vi "TSM Initialise Global (Main Sequence).vi"(0 "TSM context":T1) -> (15 "error out":errorcluster)   [LabVIEW 2019]
uses:
  <vilib>/NI_TestStand_SemiconductorModule/NI_TestStand_Semiconductor_Module.lvlibp/PinMap/General/SemiconductorModuleContext.ctl
  Common/Instrument Control/DCPower/TSM/TSM SSC DCPower.ctl
  <vilib>/NI_TestStand_SemiconductorModule/NI_TestStand_Semiconductor_Module.lvlibp/PinMap/PinQueryContext/MultiplePinMultipleSessionQueryContext/MultiplePinMultipleSessionQueryContext.lvclass
  Common/Instrument Control/DCPower/SSC DCPower/SSC DCPower.ctl
  Common/Instrument Control/Shared SubVIs/TSM Pin Abstraction/TSM Pin Information.ctl
  Common/Instrument Control/Shared SubVIs/TSM Pin Abstraction/TSM Pin Type Identifier.ctl
  Common/Instrument Control/Shared SubVIs/TSM Pin Abstraction/TSM Expanded Pin Information.ctl
  Common/Instrument Control/Relay/Pin Map/TSM Relay.ctl
  Common/Instrument Control/DAQmx/Pin Map/TSM DAQmx Multi-Task.ctl
  Common/Instrument Control/DAQmx/Pin Map/SSC DAQmx.ctl
  TSM Context Data Access/TSM Context Data Access.lvclass/TSM Context Data Access.ctl
  TSM Context Data Access/Public/Properties/D1 - Write.vi
  TSM Context Data Access/Public/Properties/G4 - Write.vi
  TSM Context Data Access/Public/Properties/G8 - Write.vi
  TSM Context Data Access/Public/Properties/G9 - Write.vi
  TSM Context Data Access/Public/Properties/I0 - Write.vi
  TSM Context Data Access/Public/Properties/L - Write.vi
  TSM Context Data Access/Public/Properties/L0 - Write.vi
  TSM Context Data Access/Public/Properties/L1 - Write.vi
  TSM Context Data Access/Public/Properties/L7 - Write.vi
  TSM Context Data Access/Public/Properties/L2 - Write.vi
  TSM Context Data Access/Public/Properties/L3 - Write.vi
  TSM Context Data Access/Public/Properties/L4 - Write.vi
  TSM Context Data Access/Public/Properties/L5 - Write.vi
  TSM Context Data Access/Public/Properties/MODE1 - Write.vi
  TSM Context Data Access/Public/Properties/F0 - Write.vi
  TSM Context Data Access/Public/Properties/F1 - Write.vi
  TSM Context Data Access/Public/Properties/F2 - Write.vi
  TSM Context Data Access/Public/Properties/F3 - Write.vi
  TSM Context Data Access/Public/Properties/F4 - Write.vi
  TSM Context Data Access/Public/Properties/F5 - Write.vi
  TSM Context Data Access/Public/Properties/F7 - Write.vi
  TSM Context Data Access/Public/Properties/F8 - Write.vi
  TSM Context Data Access/Public/Properties/F9 - Write.vi
  TSM Context Data Access/Public/Properties/Q1 - Write.vi
  TSM Context Data Access/Public/Properties/Q2 - Write.vi
  TSM Context Data Access/Public/Properties/Q3 - Write.vi
  TSM Context Data Access/Public/Properties/Q4 - Write.vi
  TSM Context Data Access/Public/Properties/Q5 - Write.vi
  TSM Context Data Access/Public/Properties/Q6 - Write.vi
  TSM Context Data Access/Public/Properties/Q7 - Write.vi
  TSM Context Data Access/Public/Properties/Q8 - Write.vi
  TSM Context Data Access/Public/Properties/Q9 - Write.vi
  TSM Context Data Access/Public/Properties/DNUM - Read.vi
  <vilib>/NI_TestStand_SemiconductorModule/NI_TestStand_Semiconductor_Module.lvlibp/PinMap/Site and Global Data/SetSiteData.vi
  <vilib>/NI_TestStand_SemiconductorModule/NI_TestStand_Semiconductor_Module.lvlibp/PinMap/Site and Global Data/SetGlobalData.vi
  <vilib>/NI_TestStand_SemiconductorModule/NI_TestStand_Semiconductor_Module.lvlibp/PinMap/Site and Global Data/GetGlobalData.vi
  <vilib>/NI_TestStand_SemiconductorModule/NI_TestStand_Semiconductor_Module.lvlibp
  TSM Context Data Access/TSM Context Data Access.lvclass
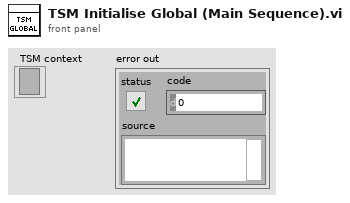
[diagram p1: front panel]
types:
  T1 = typedef "NI_TestStand_Semiconductor_Module.lvlibp/SemiconductorModuleContext.ctl" = refnum<k7>
  T2 = cluster{"unloaded12VRLY":dbl[], "vdiode":dbl[], "RelayDrop":dbl[][]}
  T3 = typedef "TSM SSC DCPower.ctl" = cluster{"Pin Query Context":refnum<class "MultiplePinMultipleSessionQueryContext.lvclass">, "SSC":T4[], "Site Numbers":i32[], "Pins":T5[], "Pins Expanded":T7[]}
  T4 = typedef "SSC DCPower.ctl" = cluster{"Session":refnum<k15>, "Chan":string, "Channel List":string}
  T5 = typedef "TSM Pin Information.ctl" = cluster{"Pin":tag, "Type":T6, "Count":i32}
  T6 = typedef "TSM Pin Type Identifier.ctl" = enum8{"DUT Pin", "System Pin", "Pin Group", "Not Determined"}
  T7 = typedef "TSM Expanded Pin Information.ctl" = cluster{"Pin":tag, "Type":T6, "Index":i32}
  T8 = typedef "TSM Relay.ctl" = cluster{"TSM Context":T1, "Relays":tag[]}
  T9 = typedef "TSM DAQmx Multi-Task.ctl" = cluster{"Pin Query Context":refnum<class "MultiplePinMultipleSessionQueryContext.lvclass">, "SSC":T10[], "Site Numbers":i32[]}
  T10 = typedef "SSC DAQmx.ctl" = cluster{"DAQmx Task ":refnum<k21>, "Channels":string, "Channel Lists":string}
  T11 = cluster{"Number Of Sites":i32, "Site Numbers":i32[], "RLY12V_MEAS":T3, "Relays Filtered Pins":string[], "Relay Pin Sessions":T8[], "UDB_EN":T9}
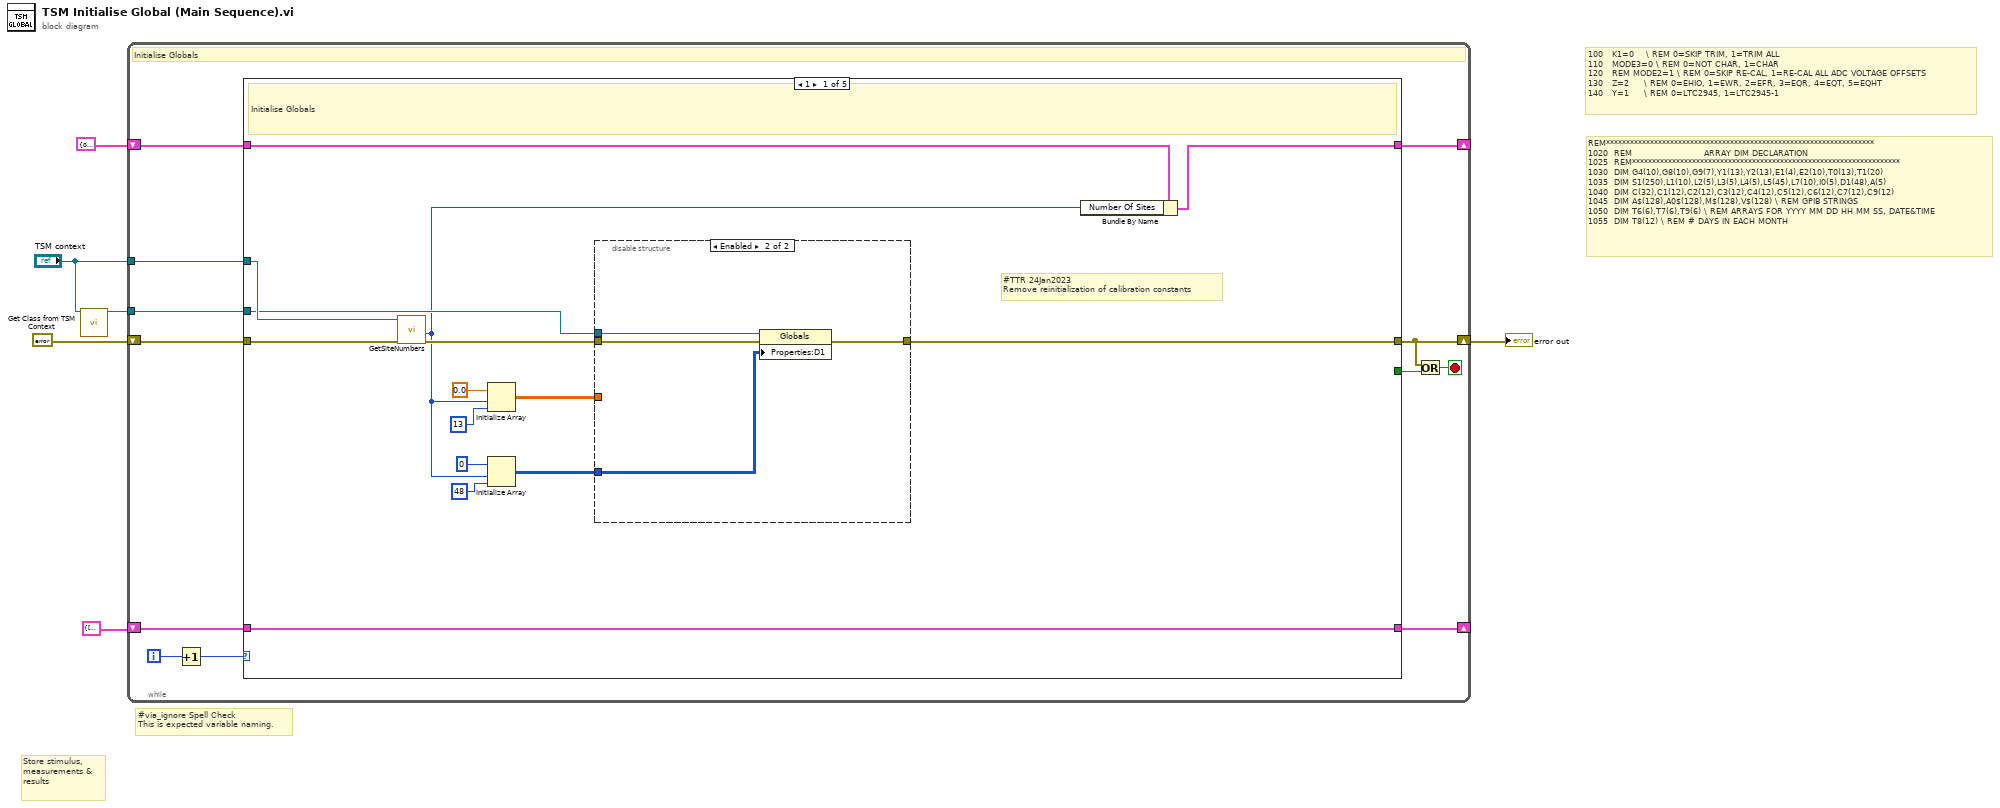
[diagram p0: block diagram]
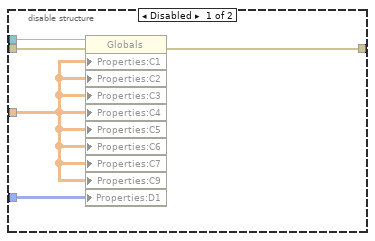
[diagram p2: hidden frame]
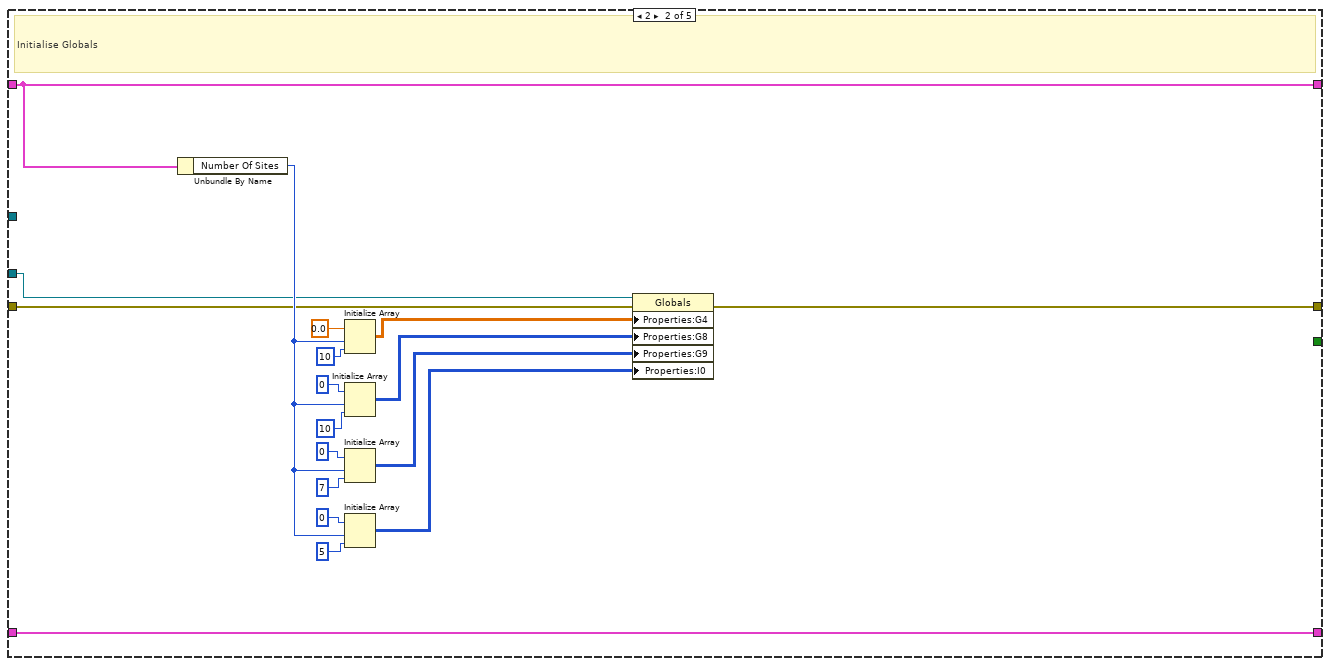
[diagram p3: hidden frame]
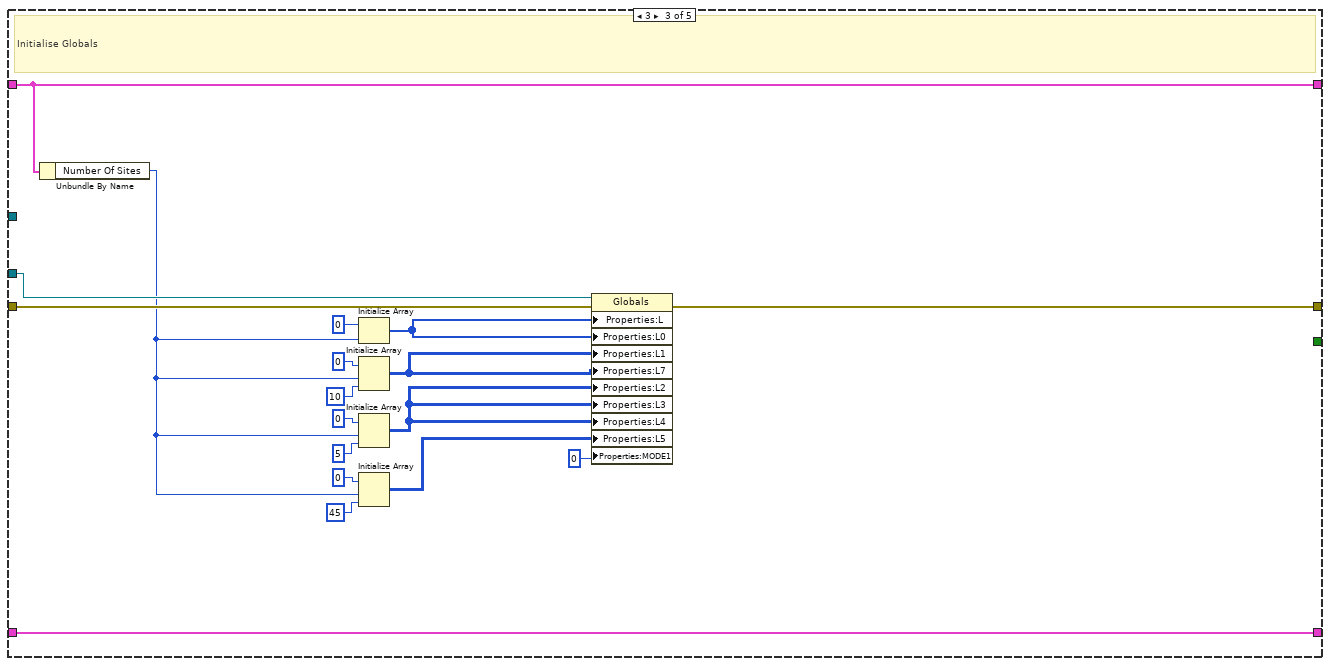
[diagram p4: hidden frame]
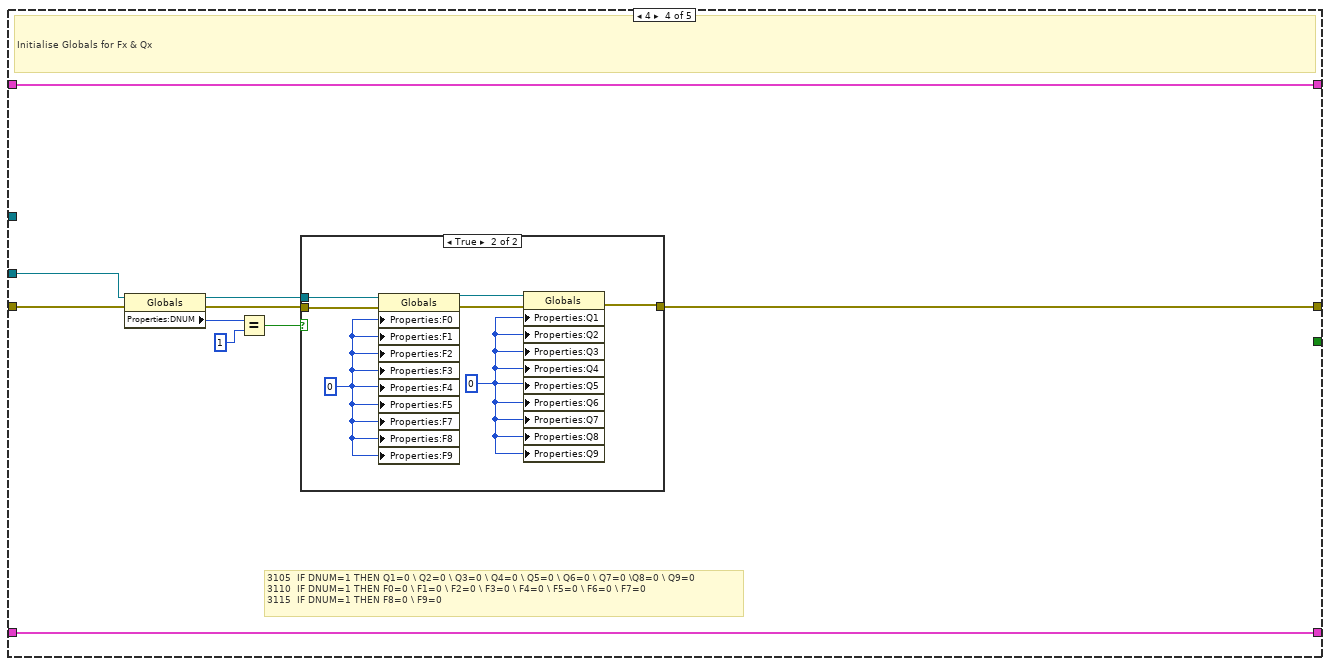
[diagram p5: hidden frame]
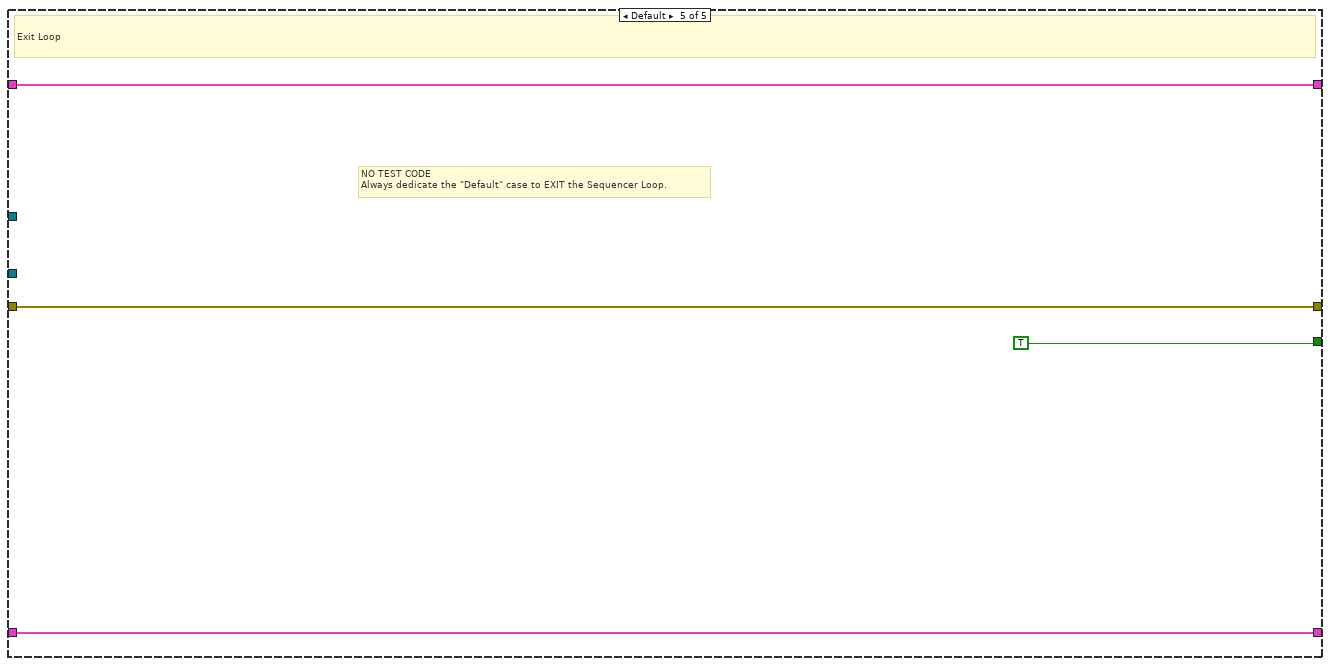
[diagram p7: hidden frame]
diagram:
  # "100   K1=0    \\ REM 0=SKIP TRIM, 1=TRIM ALL\n110   MODE3=0 \\ REM 0=NOT CHAR, 1=CHAR\n120   REM MODE2=1 \\ REM 0=SKIP RE-CAL, 1=RE-CAL ALL ADC VOLTAGE OFFSETS\n130   Z=2     \\ REM 0=EHIO, 1=EWR, 2=EFR, 3=EQR, 4=EQT, 5=EQHT\n140   Y=1     \\ REM 0=LTC2945, 1=LTC2945-1"
  # "REM*******************************************************************\n1020  REM                        ARRAY DIM DECLARATION\n1025  REM*******************************************************************\n1030  DIM G4(10),G8(10),G9(7),Y1(13),Y2(13),E1(4),E2(10),T0(13),T1(20)\n1035  DIM S1(250),L1(10),L2(5),L3(5),L4(5),L5(45),L7(10),I0(5),D1(48),A(5)\n1040  DIM C(32),C1(12),C2(12),C3(12),C4(12),C5(12),C6(12),C7(12),C9(12)\n1045  DIM A$(128),A0$(128),M$(128),V$(128) \\ REM GPIB STRINGS\n1050  DIM T6(6),T7(6),T9(6) \\ REM ARRAYS FOR YYYY MM DD HH MM SS, DATE&TIME\n1055  DIM T8(12) \\ REM # DAYS IN EACH MONTH"
  # "#via_ignore Spell Check\nThis is expected variable naming."
  # "Store stimulus, measurements & results"
  n1 = call "Get Class from TSM Context.vi"("TSM Context"="TSM context") -> ("Global Memory Class"=w2:refnum<class "TSM Context Data Access.lvclass">)  [unwired: 14 in]
  n2 = while {
    shift-right: [w10] -> w6
    shift-left: errorcluster {"status"=FALSE, "code"=0, "source"=""} ("error in") -> [w17]
    tunnel: "TSM context" -> [w15]
    shift-right: [w12] -> _
    shift-left: T11 {"Number Of Sites"=0, "Site Numbers"=[], "RLY12V_MEAS"={"Pin Query Context"=refnum, "SSC"=[], "Site Numbers"=[], "Pins"=[], "Pins Expanded"=[]}, "Relays Filtered Pins"=[], "Relay Pin Sessions"=[], "UDB_EN"={"Pin Query Context"=refnum, "SSC"=[], "Site Numbers"=[]}} -> [w13]
    shift-right: [w9] -> _
    shift-left: T2 {"unloaded12VRLY"=[], "vdiode"=[], "RelayDrop"=[]} -> [w8]
    tunnel: w2 -> [w7]
    i -> [w18]
    stop <- w11 stop-if-true
    # "Initialise Globals"
    n3 = Increment(x=w18) -> (x+1=w16:i32)
    n4 = case shown="1" w16 {
      tunnel: [w24 w58 w61 w88 w99] -> w10
      tunnel: w17 -> [w33 w44 w77 w86 w99]
      tunnel: w15 -> [w32 _ _ _ _]
      tunnel: [_ _ _ _ TRUE] -> w14
      tunnel: w13 -> [w29 w59 w76 w79 w98]
      tunnel: [w28 w59 w76 w79 w98] -> w12
      tunnel: [w23 w60 w78 w87 w97] -> w9
      tunnel: w8 -> [w23 w60 w78 w87 w97]
      tunnel: w7 -> [w30 w43 w75 w85 _]
      frame 1 {
        # "#TTR 24Jan2023\nRemove reinitialization of calibration constants"
        # "Initialise Globals"
        n5 = call <vilib>:"GetSiteNumbers.vi"("error in (no error)"=w33, "Semiconductor Module Context"=w32) -> ("error out"=w31:errorcluster, "Number Of Sites"=w19:i32)  [unwired: 6 in, 2 out]
        n6 = Initialize Array(0.0 ("element"), w19, 13 ("dimension size")) -> (w25:dbl[][])
        n7 = Initialize Array(u32 0 ("element"), w19, 48 ("dimension size")) -> (w20:u32[][])
        n8 = disable-structure shown="Enabled" {
          disable-tunnel: w31 -> [w38 w42]
          disable-tunnel: w30 -> [w37 w41]
          disable-tunnel: w25 -> [w36 _]
          disable-tunnel: [w35 w40] -> w24
          disable-tunnel: w20 -> [w34 w39]
          frame Disabled {
            n9 = property class="Globals"(reference=w37, error in=w38, "Properties:C1"=w36, "Properties:C2"=w36, "Properties:C3"=w36, "Properties:C4"=w36, "Properties:C5"=w36, "Properties:C6"=w36, "Properties:C7"=w36, "Properties:C9"=w36, "Properties:D1"=w34) -> (error out=w35:errorcluster)  [unwired: 1 out]
          }
          frame Enabled {
            n10 = property class="Globals"(reference=w41, error in=w42, "Properties:D1"=w39) -> (error out=w40:errorcluster)  [unwired: 1 out]
          }
        }
        n11 = Bundle By Name(cluster=w29, "Number Of Sites"=w19) -> (w28:T11)
      }
      frame 2 {
        # "Initialise Globals"
        n12 = Unbundle By Name(w59) -> ("Number Of Sites"=w46:i32)
        n13 = Initialize Array(0.0 ("element"), w46, 10 ("dimension size")) -> (w45:dbl[][])
        n14 = Initialize Array(0 ("element"), w46, 10 ("dimension size")) -> (w53:i32[][])
        n15 = Initialize Array(0 ("element"), w46, 7 ("dimension size")) -> (w50:i32[][])
        n16 = Initialize Array(u32 0 ("element"), w46, 5 ("dimension size")) -> (w47:u32[][])
        n17 = property class="Globals"(reference=w43, error in=w44, "Properties:G4"=w45, "Properties:G8"=w53, "Properties:G9"=w50, "Properties:I0"=w47) -> (error out=w58:errorcluster)  [unwired: 1 out]
      }
      frame 3 {
        # "Initialise Globals"
        n18 = Unbundle By Name(w76) -> ("Number Of Sites"=w62:i32)
        n19 = Initialize Array(u32 0 ("L"), w62) -> (w71:u32[])
        n20 = Initialize Array(u32 0 ("element"), w62, 10 ("dimension size")) -> (w64:u32[][])
        n21 = Initialize Array(u32 0 ("element"), w62, 5 ("dimension size")) -> (w68:u32[][])
        n22 = Initialize Array(u32 0 ("element"), w62, 45 ("dimension size")) -> (w65:u32[][])
        n23 = property class="Globals"(reference=w75, error in=w77, "Properties:L"=w71, "Properties:L0"=w71, "Properties:L1"=w64, "Properties:L7"=w64, "Properties:L2"=w68, "Properties:L3"=w68, "Properties:L4"=w68, "Properties:L5"=w65, "Properties:MODE1"=i8 0 ("MODE1")) -> (error out=w61:errorcluster)  [unwired: 1 out]
      }
      frame 4 {
        # "3105  IF DNUM=1 THEN Q1=0 \\ Q2=0 \\ Q3=0 \\ Q4=0 \\ Q5=0 \\ Q6=0 \\ Q7=0 \\Q8=0 \\ Q9=0\n3110  IF DNUM=1 THEN F0=0 \\ F1=0 \\ F2=0 \\ F3=0 \\ F4=0 \\ F5=0 \\ F6=0 \\ F7=0\n3115  IF DNUM=1 THEN F8=0 \\ F9=0"
        # "Initialise Globals for Fx & Qx"
        n24 = property class="Globals"(reference=w85, error in=w86) -> (reference out=w84:refnum<class "TSM Context Data Access.lvclass">, error out=w83:errorcluster, "Properties:DNUM"=w82:i32)
        n25 = Equal?(x=w82, y=1) -> (x = y?=w80:bool)
        n26 = case shown="True" w80 {
          tunnel: [w89 w92] -> w88
          tunnel: w84 -> [_ w96]
          tunnel: w83 -> [w89 w95]
          frame False {
          }
          frame True {
            w90 = 0 ("F0")
            w91 = 0 ("F0")
            n27 = property class="Globals"(reference=w96, error in=w95, "Properties:F0"=w91, "Properties:F1"=w91, "Properties:F2"=w91, "Properties:F3"=w91, "Properties:F4"=w91, "Properties:F5"=w91, "Properties:F7"=w91, "Properties:F8"=w91, "Properties:F9"=w91) -> (reference out=w93:refnum<class "TSM Context Data Access.lvclass">, error out=w94:errorcluster)
            n28 = property class="Globals"(reference=w93, error in=w94, "Properties:Q1"=w90, "Properties:Q2"=w90, "Properties:Q3"=w90, "Properties:Q4"=w90, "Properties:Q5"=w90, "Properties:Q6"=w90, "Properties:Q7"=w90, "Properties:Q8"=w90, "Properties:Q9"=w90) -> (error out=w92:errorcluster)  [unwired: 1 out]
          }
        }
      }
      frame Default {
        # "NO TEST CODE\nAlways dedicate the \"Default\" case to EXIT the Sequencer Loop."
        # "Exit Loop"
      }
    }
    n29 = Or(x=w10, y=w14) -> (x .or. y?=w11:bool)
  }
  "error out" <- w6
